vi "filterAndRRPeaksDet.vi"(9 "fs":dbl, 10 "ECG1":dbl[](array[numeric])) -> (0 "Filtered ECG1":dbl[](array[numeric]), 1 "Amplitudes":dbl[](array[numeric]), 2 "Locations":dbl[](array[numeric]), 3 "# peaks":dbl, 11 "Time":dbl[](array[numeric]))   [LabVIEW 2025]
uses:
  <vilib>/Analysis/3filter.llb/Butterworth Filter (DBL).vi
  <vilib>/Analysis/NI_AALBase.lvlib
  <vilib>/Analysis/NI_AAL_SigProc.lvlib
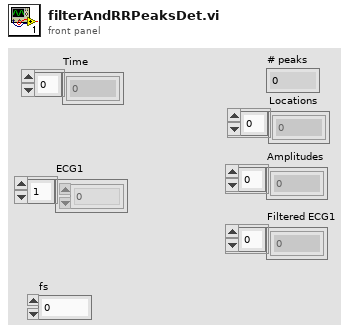
[diagram p1: front panel]
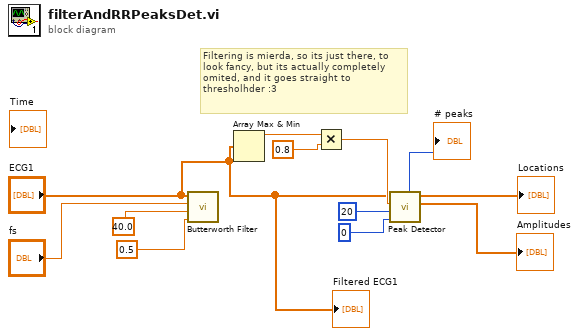
[diagram p0: block diagram]
diagram:
  # "Filtering is mierda, so its just there, to look fancy, but its actually completely omited, and it goes straight to thresholhder :3"
  n1 = call-poly <vilib>:"Butterworth Filter.vi"("low cutoff freq: fl"=0.5, "high cutoff freq: fh"=40.0, "sampling freq: fs"="fs", "X"="ECG1") -> ()  [unwired: 4 in, 2 out]
  n2 = Array Max & Min(array="ECG1") -> (max value=w9:dbl)  [unwired: 3 out]
  n3 = Multiply(x=w9, y=0.8) -> (x*y=w7:dbl)
  n4 = call <vilib>:"Peak Detector.vi"("peaks/valleys"=0, "width"=20, "threshold"=w7, "X"="ECG1") -> ("Amplitudes"=→"Amplitudes":dbl[], "Locations"=→"Locations":dbl[], "# found"=→"# peaks":i32)  [unwired: 3 in, 2 out]
  "Filtered ECG1" <- "ECG1"
